vi "Persistence.vi"() -> ()   [LabVIEW 2020]
uses:
  d94e0766-a9f8-4b91-b199-a4dd9911b6b9.vi
  <vilib>/measure/NI_MABase.lvlib
panel:
  out "Palette 2":u32[](array[colorbox])
  in  "Signal Type 2":enum16{"Sine", "Gauss", "Sine + Gauss"}(ring)=enum."Sine + Gauss"
  out "Available History Buffer Depth 2":i32=17
  out "Available History Buffer Depth 1":i32=17
  in  "Combine signals to Signal 2":enum16{"None", "Add 1 and 2"}(ring)
  in  "Signal Type 1":enum16{"Sine", "Gauss", "Sine + Gauss"}(ring)=enum."Sine + Gauss"
  in  "frequency 2":dbl=3.0 format="%0.2p"
  in  "amplitude 2":dbl=0.75 format="%0.2p"
  in  "phase 2 [deg]":dbl=-2.0
  in  "sampling info 2":cluster{"Fs":dbl, "#s":dbl}={"Fs"=1000.0, "#s"=1000.0} {"Fs" format="%.2p"}
  out "Palette 1":u32[](array[colorbox])
  in  "NumOfPlots (History)":u32=17
  out "Combined Plots":waveform(dbl)[](graph)
  in  "frequency":dbl=10.0 format="%0.2p"
  in  "amplitude":dbl=1.0 format="%0.2p"
  in  "phase [deg]":dbl=3.0
  in  "sampling info":cluster{"Fs":dbl, "#s":dbl}={"Fs"=1000.0, "#s"=1000.0} {"Fs" format="%.2p"}
  in  "stop":bool
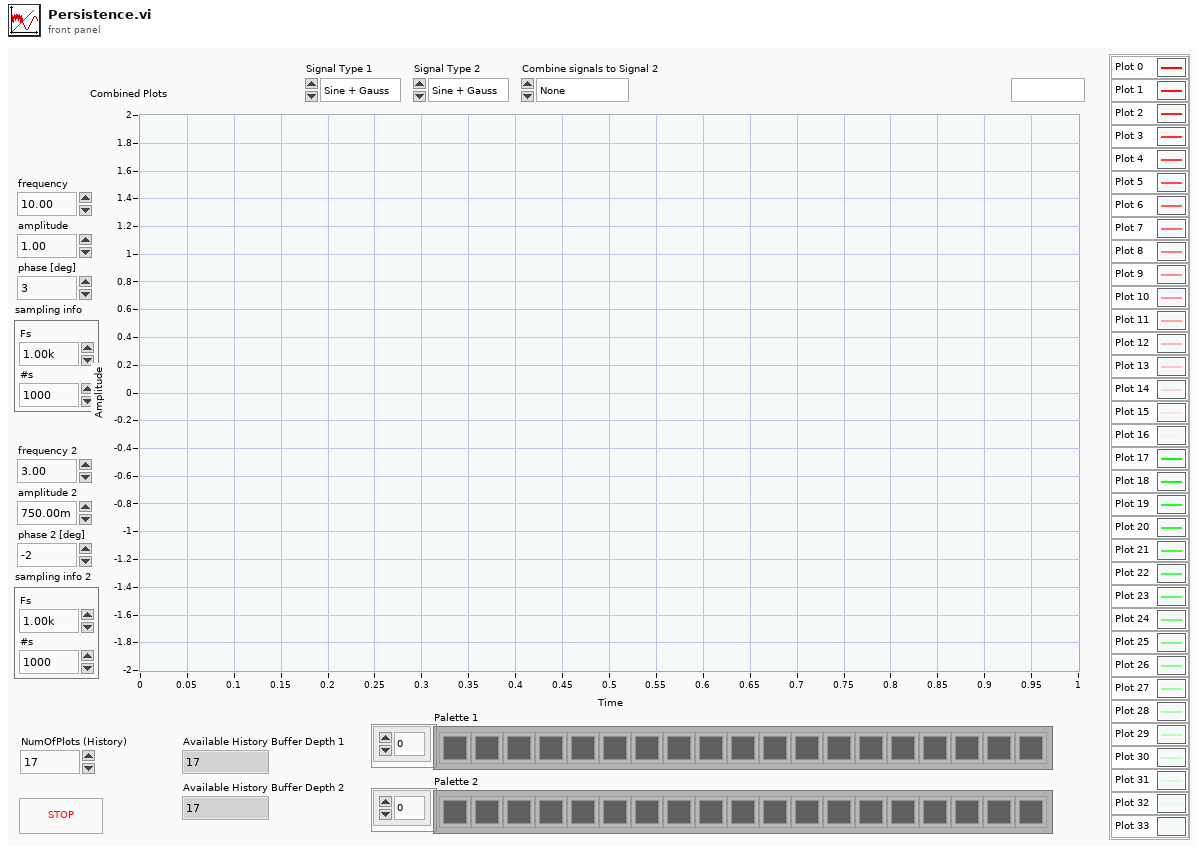
[diagram p1: front panel]
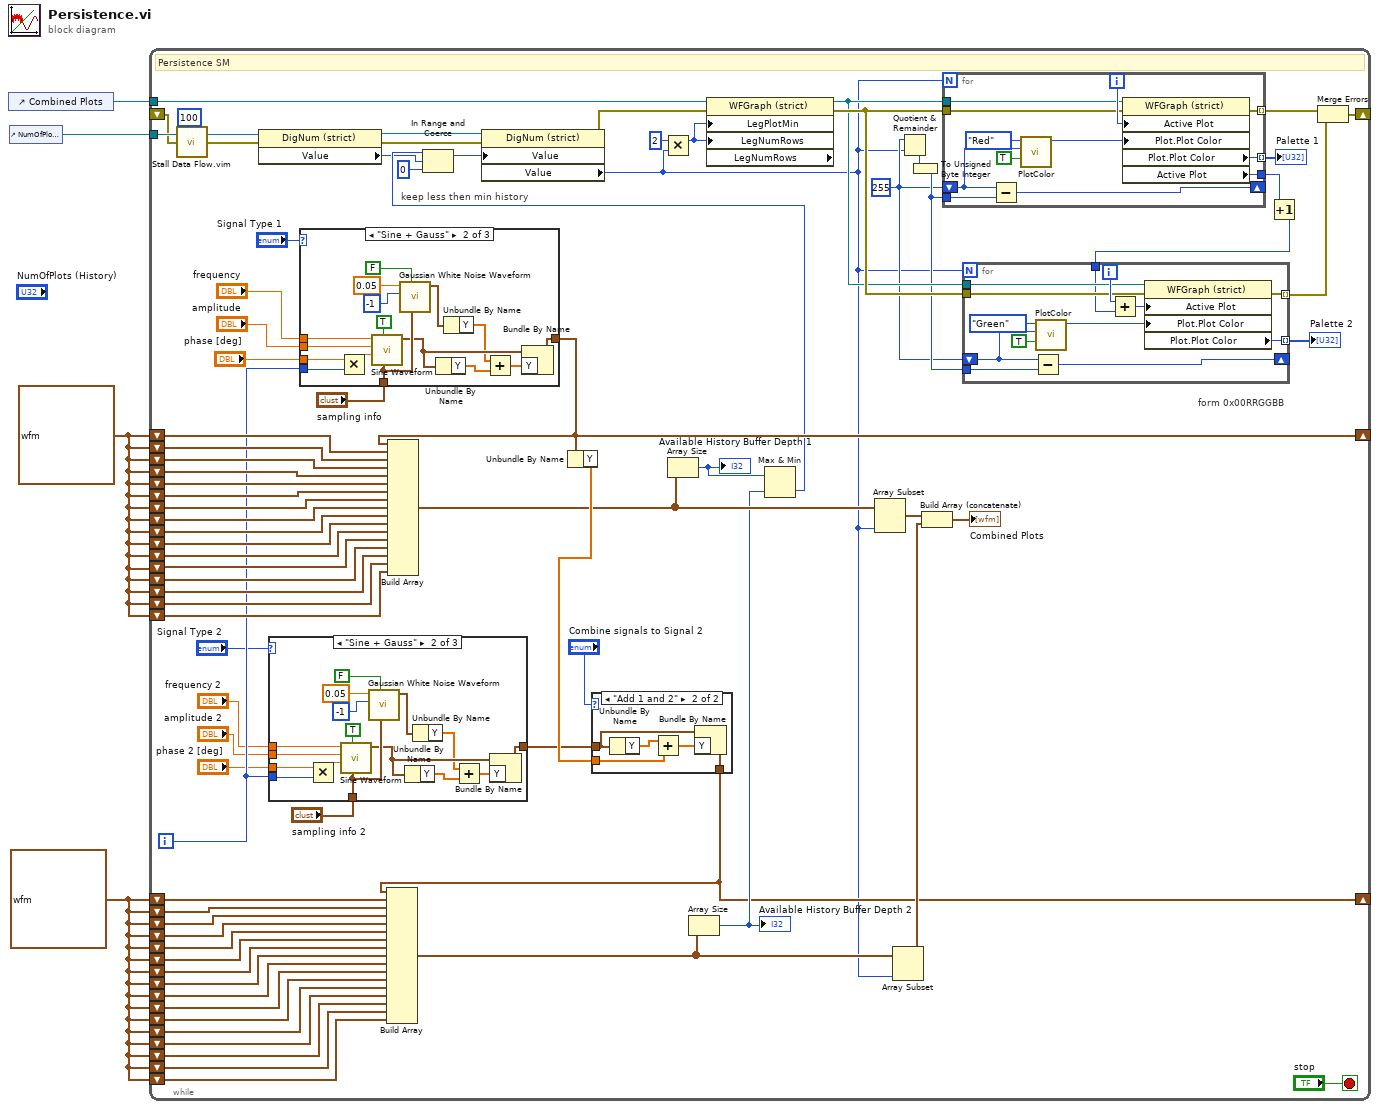
[diagram p0: block diagram]
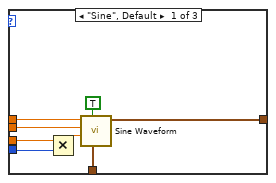
[diagram p2: hidden frame]
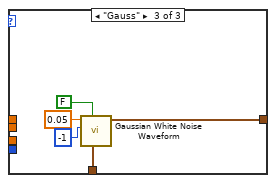
[diagram p3: hidden frame]
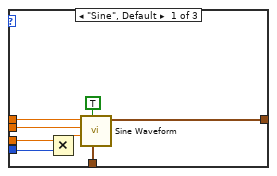
[diagram p5: hidden frame]
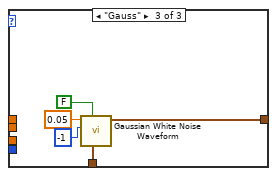
[diagram p6: hidden frame]
diagram:
  w4 = waveform(dbl) {"t0"=timestamp(0 s since 1904-01-01), "dt"=1.0, "Y"=[]} ("signal out")
  w3 = waveform(dbl) {"t0"=timestamp(0 s since 1904-01-01), "dt"=1.0, "Y"=[]} ("signal out")
  n1 = control-ref of="Combined Plots"() -> (w2:refnum<vi>)
  n2 = control-ref of="NumOfPlots (History)"() -> (w1:refnum<vi>)
  n3 = while {
    shift-right: [w46] -> _
    shift-left: w3 -> [w76]
    shift-left: w3 -> [w85]
    shift-left: w3 -> [w84]
    shift-left: w3 -> [w83]
    shift-left: w3 -> [w82]
    shift-left: w3 -> [w81]
    shift-left: w3 -> [w80]
    shift-left: w3 -> [w79]
    shift-left: w3 -> [w78]
    shift-left: w3 -> [w77]
    shift-left: w3 -> [w75]
    shift-left: w3 -> [w74]
    shift-right: [w27] -> _
    shift-left: w4 -> [w70]
    shift-left: w4 -> [w69]
    shift-left: w4 -> [w68]
    shift-left: w4 -> [w67]
    shift-left: w4 -> [w66]
    shift-left: w4 -> [w65]
    shift-left: w4 -> [w64]
    shift-left: w4 -> [w63]
    shift-left: w4 -> [w62]
    shift-left: w4 -> [w61]
    shift-left: w4 -> [w60]
    shift-left: w4 -> [w59]
    shift-left: w4 -> [w58]
    shift-left: w4 -> [w57]
    shift-left: w3 -> [w43]
    shift-left: w3 -> [w42]
    shift-left: w3 -> [w41]
    shift-left: w4 -> [w30]
    shift-left: w4 -> [w29]
    shift-left: w3 -> [w28]
    tunnel: w2 -> [w26]
    tunnel: w1 -> [w25]
    shift-right: [w8] -> _
    shift-left: _ -> [w7]
    i -> [w16]
    stop <- "stop" stop-if-true
    w52 = u8 255
    # "keep less then min history"
    # "form 0x00RRGGBB"
    # "Persistence SM"
    n4 = call "Stall Data Flow.vim"("value in"=w7, "milliseconds to wait"=u32 100) -> ("value out"=w6:errorcluster)  [unwired: 1 out]
    n5 = property class="DigNum (strict)"(reference=w25, error in=w6) -> (reference out=w32:refnum<vi>, error out=w24:errorcluster, "Value"=w33:u32)
    n6 = case shown="\"Sine + Gauss\"" "Signal Type 2" {
      tunnel: "sampling info 2" -> [w89 w102 w112]
      tunnel: w16 -> [w93 w109 _]
      tunnel: [w88 w98 w113] -> w18
      tunnel: "phase 2 [deg]" -> [w92 w108 _]
      tunnel: "amplitude 2" -> [w91 w107 _]
      tunnel: "frequency 2" -> [w90 w106 _]
      frame "Sine", Default {
        n7 = Multiply(x=w92, y=w93) -> (x*y=w94:dbl)
        n8 = call <vilib>:"Sine Waveform.vi"("sampling info"=w89, "reset signal"=TRUE, "phase"=w94, "amplitude"=w91, "frequency"=w90) -> ("signal out"=w88:waveform(dbl))  [unwired: 5 in, 1 out]
      }
      frame "Sine + Gauss" {
        n9 = Multiply(x=w108, y=w109) -> (x*y=w110:dbl)
        n10 = call <vilib>:"Sine Waveform.vi"("sampling info"=w102, "reset signal"=TRUE, "phase"=w110, "amplitude"=w107, "frequency"=w106) -> ("signal out"=w99:waveform(dbl))  [unwired: 5 in, 1 out]
        n11 = call <vilib>:"Gaussian White Noise Waveform.vi"("sampling info"=w102, "reset signal"=FALSE, "seed"=-1, "standard deviation"=0.05) -> ("signal out"=w97:waveform(dbl))  [unwired: 6 in, 1 out]
        n12 = Unbundle By Name(w99) -> ("Y"=w101:dbl[])
        n13 = Unbundle By Name(w97) -> ("Y"=w96:dbl[])
        n14 = Add(x=w96, y=w101) -> (x+y=w100:dbl[])
        n15 = Bundle By Name(cluster=w99, "Y"=w100) -> (w98:waveform(dbl))
      }
      frame "Gauss" {
        n16 = call <vilib>:"Gaussian White Noise Waveform.vi"("sampling info"=w112, "reset signal"=FALSE, "seed"=-1, "standard deviation"=0.05) -> ("signal out"=w113:waveform(dbl))  [unwired: 6 in, 1 out]
      }
    }
    n17 = case shown="\"Sine + Gauss\"" "Signal Type 1" {
      tunnel: "sampling info" -> [w124 w137 w147]
      tunnel: w16 -> [w128 w144 _]
      tunnel: [w123 w133 w148] -> w46
      tunnel: "phase [deg]" -> [w127 w143 _]
      tunnel: "amplitude" -> [w126 w142 _]
      tunnel: "frequency" -> [w125 w141 _]
      frame "Sine", Default {
        n18 = Multiply(x=w127, y=w128) -> (x*y=w129:dbl)
        n19 = call <vilib>:"Sine Waveform.vi"("sampling info"=w124, "reset signal"=TRUE, "phase"=w129, "amplitude"=w126, "frequency"=w125) -> ("signal out"=w123:waveform(dbl))  [unwired: 5 in, 1 out]
      }
      frame "Sine + Gauss" {
        n20 = Multiply(x=w143, y=w144) -> (x*y=w145:dbl)
        n21 = call <vilib>:"Sine Waveform.vi"("sampling info"=w137, "reset signal"=TRUE, "phase"=w145, "amplitude"=w142, "frequency"=w141) -> ("signal out"=w134:waveform(dbl))  [unwired: 5 in, 1 out]
        n22 = call <vilib>:"Gaussian White Noise Waveform.vi"("sampling info"=w137, "reset signal"=FALSE, "seed"=-1, "standard deviation"=0.05) -> ("signal out"=w132:waveform(dbl))  [unwired: 6 in, 1 out]
        n23 = Unbundle By Name(w134) -> ("Y"=w136:dbl[])
        n24 = Unbundle By Name(w132) -> ("Y"=w131:dbl[])
        n25 = Add(x=w131, y=w136) -> (x+y=w135:dbl[])
        n26 = Bundle By Name(cluster=w134, "Y"=w135) -> (w133:waveform(dbl))
      }
      frame "Gauss" {
        n27 = call <vilib>:"Gaussian White Noise Waveform.vi"("sampling info"=w147, "reset signal"=FALSE, "seed"=-1, "standard deviation"=0.05) -> ("signal out"=w148:waveform(dbl))  [unwired: 6 in, 1 out]
      }
    }
    n28 = Build Array(w46, w76, w85, w84, w83, w82, w81, w80, w79, w78, w77, w75, w74, w43, w42, w41, w28) -> (w40:waveform(dbl)[])
    n29 = Unbundle By Name(w46) -> ("Y"=w45:dbl[])
    n30 = case shown="\"Add 1 and 2\"" "Combine signals to Signal 2" {
      tunnel: w18 -> [w117 w121]
      tunnel: [w117 w120] -> w27
      tunnel: w45 -> [_ w118]
      frame "None", Default {
      }
      frame "Add 1 and 2" {
        n31 = Unbundle By Name(w121) -> ("Y"=w122:dbl[])
        n32 = Add(x=w122, y=w118) -> (x+y=w119:dbl[])
        n33 = Bundle By Name(cluster=w121, "Y"=w119) -> (w120:waveform(dbl))
      }
    }
    n34 = Build Array(w27, w70, w69, w68, w67, w66, w65, w64, w63, w62, w61, w60, w59, w58, w57, w30, w29) -> (w38:waveform(dbl)[])
    n35 = Array Size(array=w40) -> (size(s)=w37:i32)
    "Available History Buffer Depth 1" <- w37
    n36 = Array Size(array=w38) -> (size(s)=w36:i32)
    "Available History Buffer Depth 2" <- w36
    n37 = Max & Min(x=w37, y=w36) -> (min(x,y)=w35:i32)  [unwired: 1 out]
    n38 = In Range and Coerce(upper limit=w35, x=w33, lower limit=u32 0) -> (coerced(x)=w31:u32)  [unwired: 1 out]
    n39 = property class="DigNum (strict)"(reference=w32, error in=w24, "Value"=w31) -> (error out=w23:errorcluster, "Value"=w22:u32)  [unwired: 1 out]
    n40 = Multiply(x=u32 2 ("y"), y=w22) -> (x*y=w50:u32)
    n41 = property on="Property Node" class="WFGraph (strict)" props=["LegPlotMin", "LegNumRows", "LegNumRows"](reference=w26, error in=w23, "LegPlotMin"=w50, "LegNumRows"=w50) -> (reference out=w54:refnum<vi>, error out=w55:errorcluster)  [unwired: 1 out]
    n42 = Array Subset(array=w40, length=w22) -> (w72:waveform(dbl)[])  [unwired: 1 in]
    n43 = Array Subset(array=w38, length=w22) -> (w39:waveform(dbl)[])  [unwired: 1 in]
    n44 = Quotient & Remainder(x=w52, y=w22) -> (floor(x/y)=w73:u32)  [unwired: 1 out]
    n45 = To Unsigned Byte Integer(number=w73) -> (unsigned 8bit integer=w53:u8)
    n46 = Build Array (concatenate)(w72, w39) -> (→"Combined Plots":waveform(dbl)[])
    n47 = for {
      N: w22 -> [_]
      shift-right: [w173] -> _
      shift-left: w52 -> [w167]
      tunnel: w53 -> [w174]
      tunnel: w54 -> [w172]
      tunnel: w55 -> [w171]
      tunnel: [w170] -> w71 mode=indexing
      tunnel: [w169] -> w51
      tunnel: [w168] -> w10 mode=indexing
      i -> [w176]
      n48 = Subtract(x=w167, y=w174) -> (x-y=w173:u8)
      n49 = call "PlotColor.vi"("White Palette"=TRUE, "InputColorCode"=w167, "Color"=enum16{"Red", "Green", "Blue"}."Red") -> ("Color"=w175:u32)  [unwired: 8 in]
      n50 = property on="Property Node" class="WFGraph (strict)"(reference=w172, error in=w171, "Active Plot"=w176, "Plot.Plot Color"=w175) -> (error out=w168:errorcluster, "Plot.Plot Color"=w170:u32, "Active Plot"=w169:u32)  [unwired: 1 out]
    }
    "Palette 1" <- w71
    n51 = Increment(x=w51) -> (x+1=w48:u32)
    n52 = for {
      N: w22 -> [_]
      shift-right: [w162] -> _
      shift-left: w52 -> [w153]
      tunnel: w53 -> [w163]
      tunnel: w54 -> [w161]
      tunnel: w55 -> [w160]
      tunnel: [w159] -> w11 mode=indexing
      tunnel: w48 -> [w157]
      tunnel: [w156] -> w9 mode=indexing
      i -> [w164]
      n53 = Subtract(x=w153, y=w163) -> (x-y=w162:u8)
      n54 = call "PlotColor.vi"("White Palette"=TRUE, "InputColorCode"=w153, "Color"=enum16{"Red", "Green", "Blue"}."Green") -> ("Color"=w152:u32)  [unwired: 8 in]
      n55 = Add(x=w164, y=w157) -> (x+y=w158:u32)
      n56 = property on="Property Node" class="WFGraph (strict)"(reference=w161, error in=w160, "Active Plot"=w158, "Plot.Plot Color"=w152) -> (error out=w156:errorcluster, "Plot.Plot Color"=w159:u32)  [unwired: 1 out]
    }
    "Palette 2" <- w11
    n57 = Merge Errors(w10, w9) -> (w8:errorcluster)
  }
